vi "DAQ-Data-to-File Set Enable State on Multiple Controls.vi"(10 "Enable?":bool, 11 "Controls":refnum<vi>[](array[refnum])) -> ()   [LabVIEW 2020]
doc: "Sets all the controls in the input array to the \"Enable state\" value."
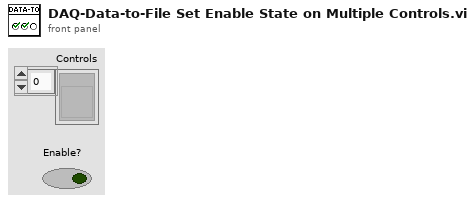
[diagram p1: front panel]
types:
  T1 = enum8{"Enabled", "Disabled", "Disabled and Grayed Out"}
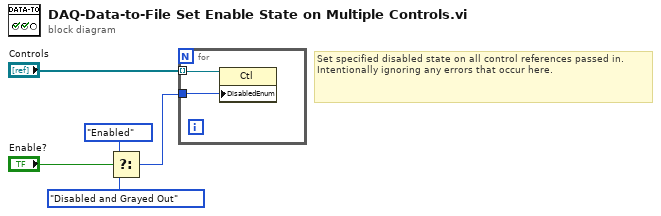
[diagram p0: block diagram]
diagram:
  # "Set specified disabled state on all control references passed in. Intentionally ignoring any errors that occur here."
  n1 = Select(t=T1."Enabled" ("Disabled"), s="Enable?", f=T1."Disabled and Grayed Out" ("Disabled")) -> (s? t:f=w3:T1)
  n2 = for {
    tunnel: "Controls" -> [w7] mode=indexing
    tunnel: w3 -> [w6]
    n3 = property class="Ctl"(reference=w7, "DisabledEnum"=w6) -> ()  [unwired: 1 in, 2 out]
  }
